vi "Dust_Type_Menu.vi"(8 "error in (no error)":errorcluster, 10 "Small?":bool, 11 "Enable":bool=TRUE) -> (0 "error out":errorcluster, 1 "Action Taken":T6(ring), 2 "Dust Properties":T3, 3 "Dust Info":T4 {"Batch" step=1; "Type" step=1; "Dust Source Builder:" items=["Keith Drake", "Nick Beaty", "Anthony Shu", "David James", "John Fontanese"]})   [LabVIEW 2013]
doc: "Displays a standard dialog box that prompts users to enter information, such as a user name and password.\n--------------------\n\nThis Express VI is configured as follows:\n\nMessage to Display to the User:Please Enter Experiment Settings Information For Database Storage.\nThe inputs are: \nNumber: Please Enter Group ID\nText Entry Box: Please Enter Tags:\nText Entry Box: Please Enter Experiment Description:"
uses:
  <vilib>/Utility/miscctls.llb/LVPointTypeDef.ctl
  <vilib>/addons/database/_DB Variant To Data/Database Variant To Data.xnode
  Controls/source_builders.ctl
  <userlib>/_OpenG.lib/array/array.llb/Remove Duplicates from 1D Array (String)__ogtk.vi
  <userlib>/_OpenG.lib/array/array.llb/Search 1D Array (String)__ogtk.vi
  <userlib>/_OpenG.lib/array/array.llb/Index 1D Array Elements (String)__ogtk.vi
  Controls/dust type.ctl
  Controls/dust_type_indicator.ctl
  Controls/Dust_list.ctl
panel:
  out "Query in Standard Format":string
  out "Maxes Array":T1(array[cluster])
  out "All Dust Types":T2[](array[typedef])
  in  "Transfer":bool caption="OK2"
  in  "Controls":T4 {"Batch" min=1 max=2 step=1; "Type" min=1 max=10 step=1; "Dust Source Builder:" items=["Keith Drake", "Nick Beaty", "Anthony Shu", "David James", "John Fontanese"]}
  in  "Create New":bool caption="OK2"
  in  "Cancel":bool
  in  "Update":bool caption="OK1"
  # "Please Enter Dust Information For Storage in the CCLDAS Database."
  # "Dust Information"
  # "Dust Information"
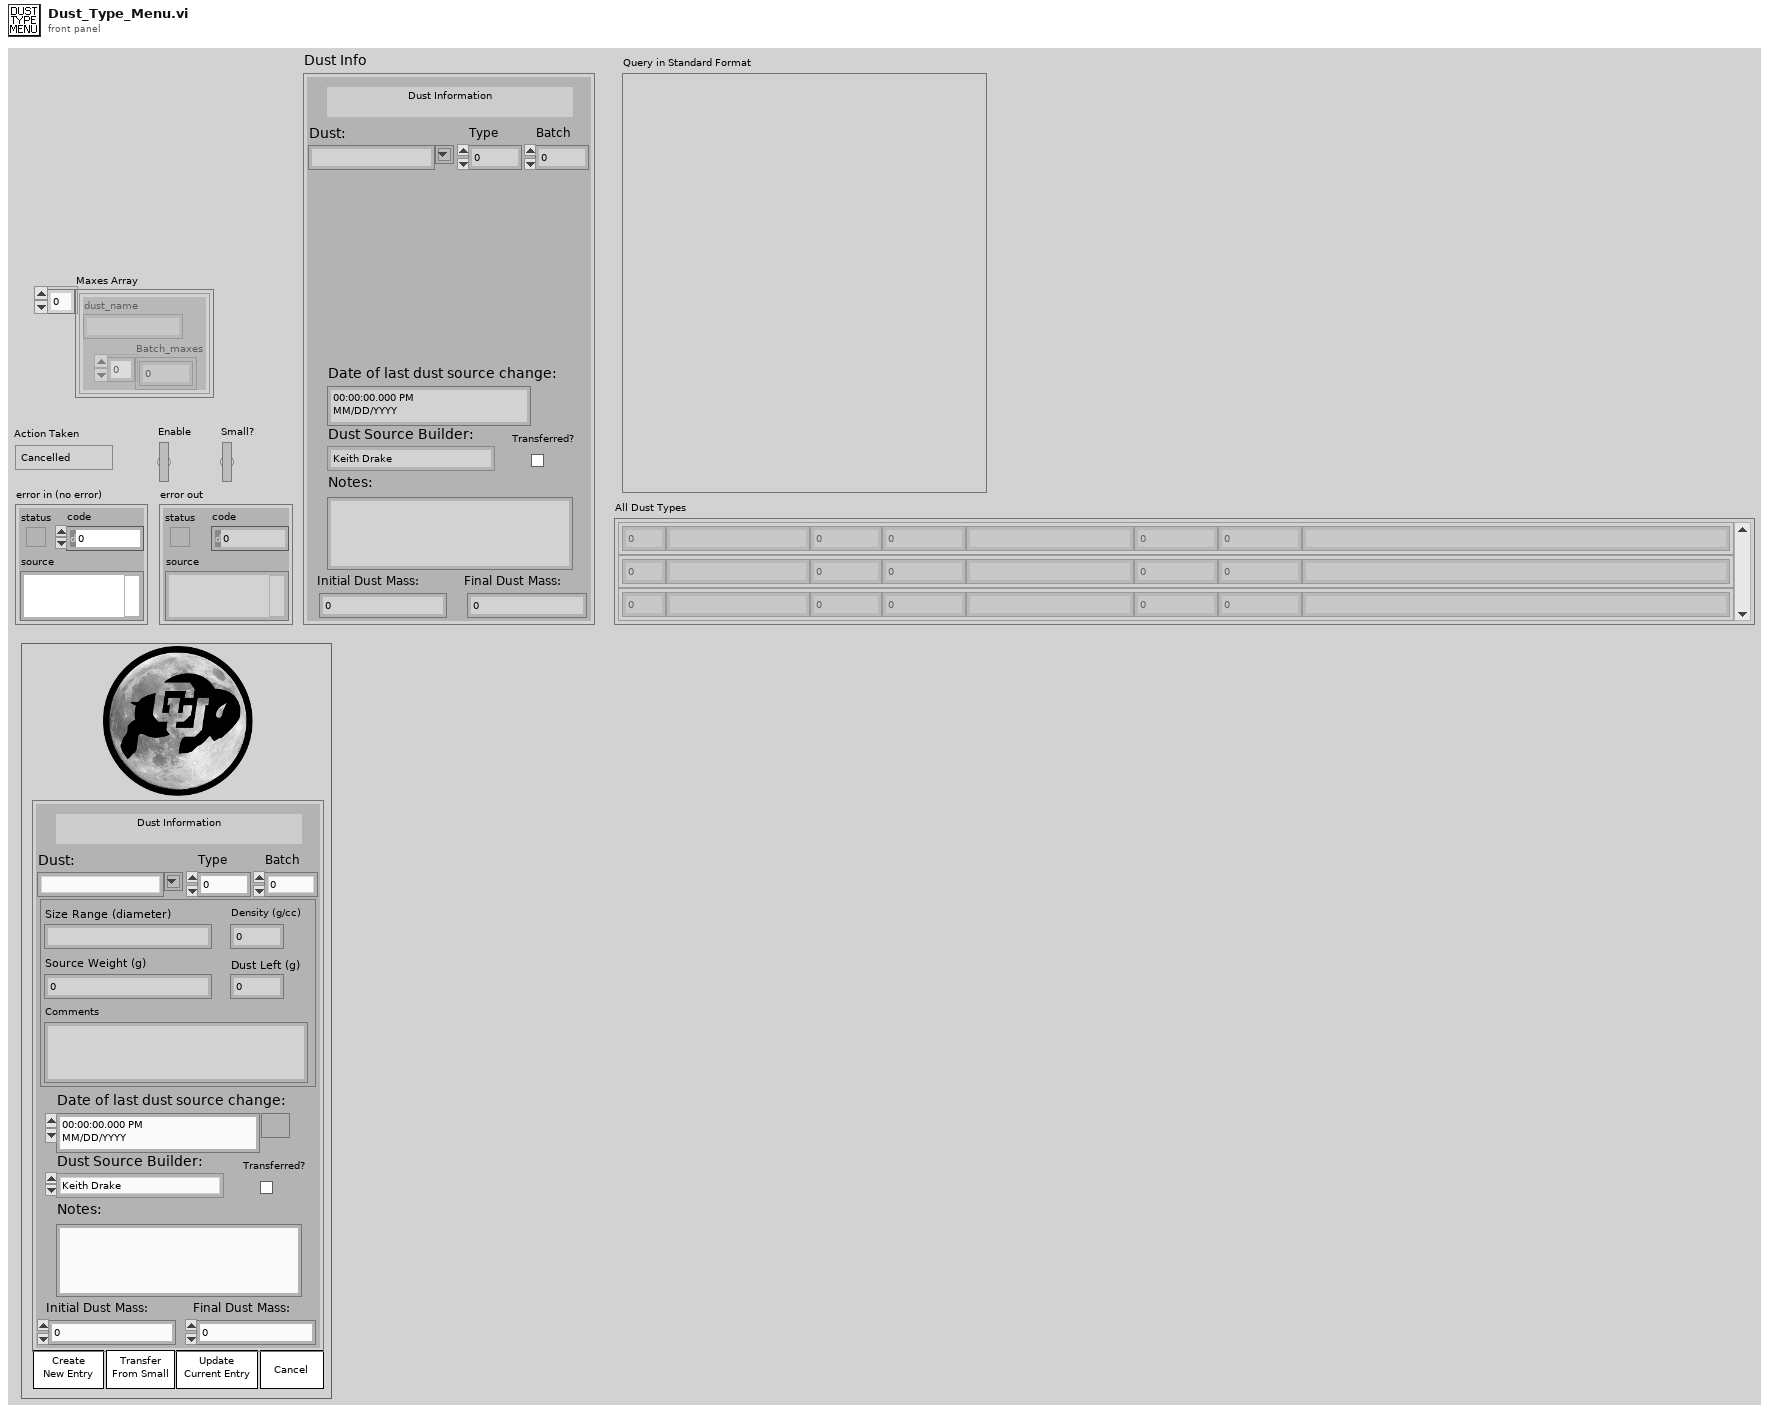
[diagram p1: front panel]
types:
  T1 = cluster{"dust_name":string, "Batch_maxes":i32[]}[]
  T2 = typedef "dust_list.ctl" = cluster{"id_dust_type":i32, "dust_name":string, "dust_density":dbl, "source_weight":dbl, "size":string, "bottle_weight":dbl, "dust_mass":dbl, "comments":string}
  T3 = typedef "dust_type_indicator.ctl" = cluster{"id_dust_type":i32, "Size Range (diameter)":string, "Density (g/cc)":dbl, "Source Weight (g)":dbl, "Dust Left (g)":dbl, "Comments":string}
  T4 = typedef "dust type.ctl" = cluster{"Dust info id":u16, "Integer Timestamp":i64, "Dust:":string, "Dust Source Builder:":T5, "Notes:":string, "Date of last dust source change:":timestamp, "Initial Dust Mass:":dbl, "Final Dust Mass:":dbl, "Type":u16, "Batch":u16, "dust type id":u16, "Transferred?":bool}
  T5 = typedef "source_builders.ctl" = u16
  T6 = enum16{"Cancelled", "New", "Updated", "Transferred"}
  T7 = enum8{"Enabled", "Disabled", "Disabled and Grayed Out"}
  T8 = typedef "LVPointTypeDef.ctl" = cluster{"Horizontal":i16, "Vertical":i16}
  T9 = enum16{"dust_name", "dust_density", "source_weight", "bottle_weight", "dust_weight"}
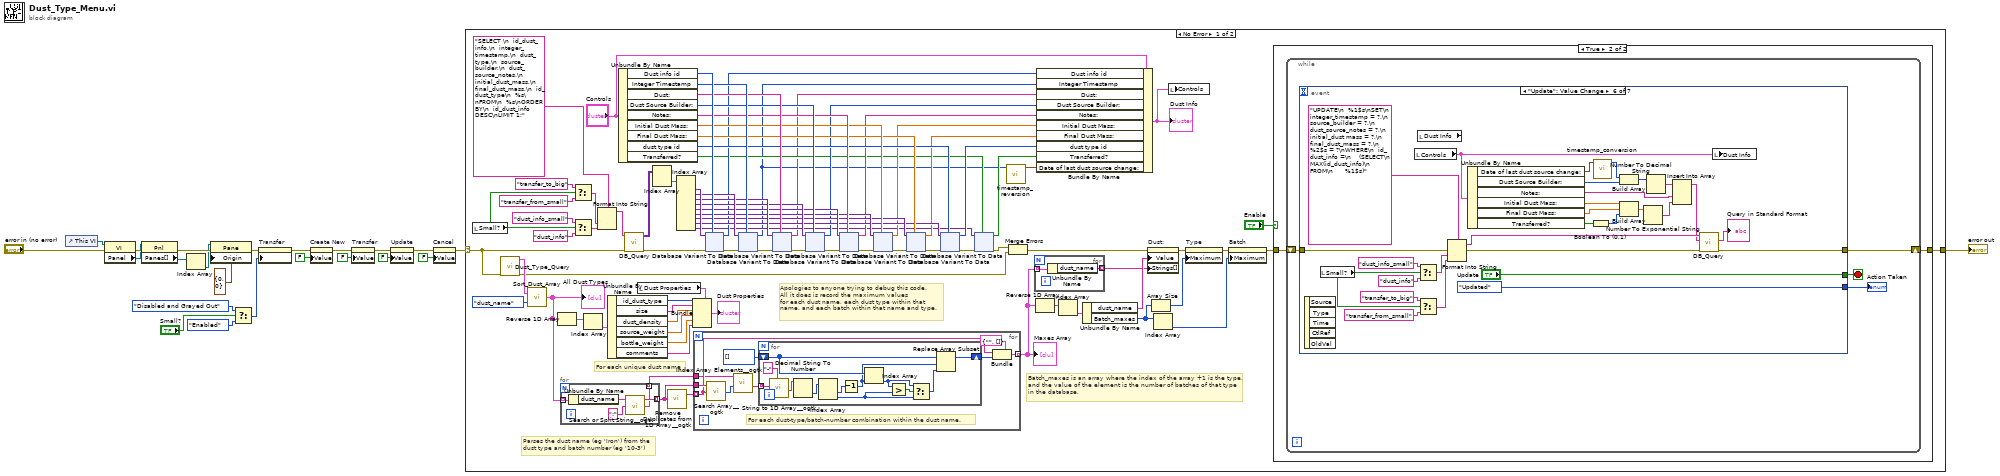
[diagram p0: block diagram]
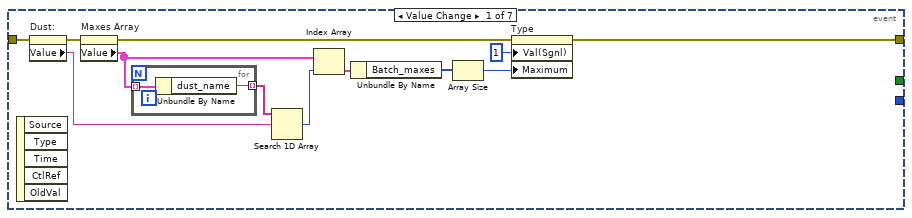
[diagram p3: hidden frame]
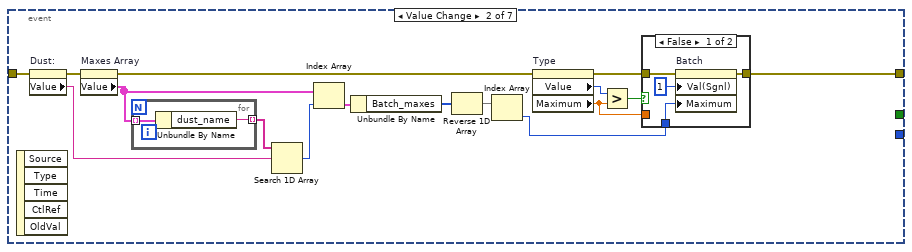
[diagram p4: hidden frame]
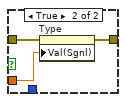
[diagram p5: hidden frame]
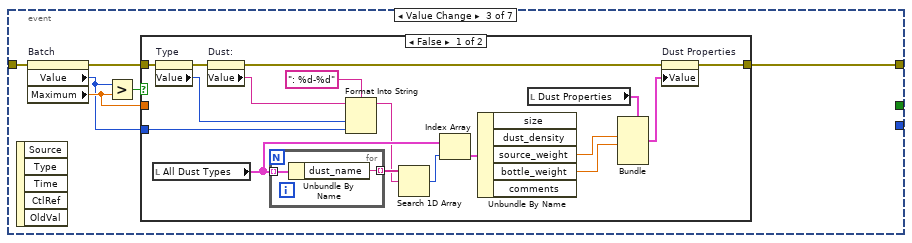
[diagram p6: hidden frame]
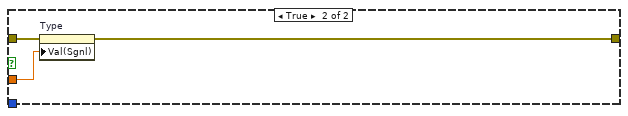
[diagram p7: hidden frame]
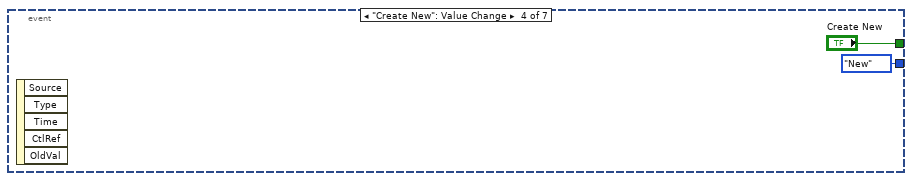
[diagram p8: hidden frame]
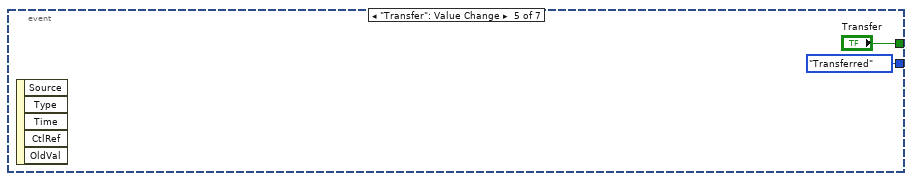
[diagram p9: hidden frame]
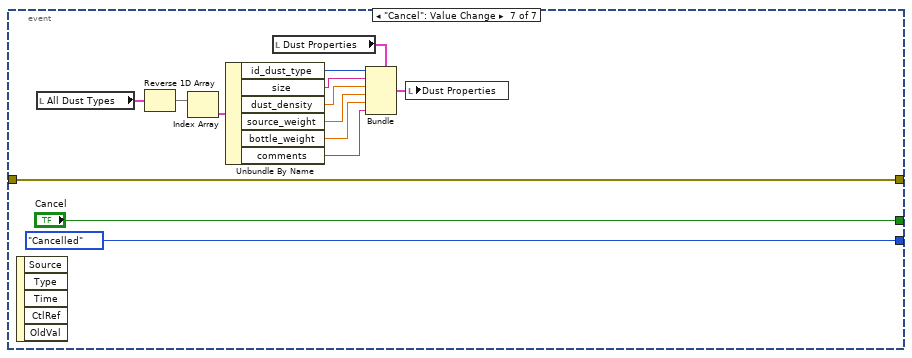
[diagram p10: hidden frame]
diagram:
  n1 = control-ref of="This VI"() -> (w22:refnum<vi>)
  n2 = property class="VI"(reference=w22, error in="error in (no error)") -> (error out=w21:errorcluster, "Panel"=w20:refnum<vi>)  [unwired: 1 out]
  n3 = property class="Pnl"(reference=w20, error in=w21) -> (error out=w19:errorcluster, "Panes[]"=w18:refnum<vi>[])  [unwired: 1 out]
  n4 = Index Array(array=w18) -> (element=w17:refnum<vi>)  [unwired: 1 in]
  n5 = property class="Pane"(reference=w17, error in=w19, "Origin"=T8 {"Horizontal"=0, "Vertical"=0}) -> (error out=w10:errorcluster)  [unwired: 1 out]
  n6 = Select(t=T7."Disabled and Grayed Out" ("Disabled"), s="Small?", f=T7."Enabled" ("Disabled")) -> (s? t:f=w13:T7)
  n7 = property on="Transfer" class="Bool (strict)"(error in=w10, "DisabledEnum"=w13) -> (error out=w5:errorcluster)  [unwired: 1 in, 1 out]
  n8 = property on="Create New" class="Bool (strict)"(error in=w5, "Value"=FALSE ("Create New")) -> (error out=w7:errorcluster)  [unwired: 1 in, 1 out]
  n9 = property on="Transfer" class="Bool (strict)"(error in=w7, "Value"=FALSE ("Transfer")) -> (error out=w9:errorcluster)  [unwired: 1 in, 1 out]
  n10 = property on="Update" class="Bool (strict)"(error in=w9, "Value"=FALSE ("Update")) -> (error out=w8:errorcluster)  [unwired: 1 in, 1 out]
  n11 = property on="Cancel" class="Bool (strict)"(error in=w8, "Value"=FALSE ("Cancel")) -> (error out=w6:errorcluster)  [unwired: 1 in, 1 out]
  n12 = case shown="No Error" w6 {
    selector: w6 -> [w58 w544]
    tunnel: [w35 w544] -> w23
    frame No Error {
      # "Batch_maxes is an array where the index of the array +1 is the type,\nand the value of the element is the number of batches of that type\nin the database."
      # "For each unique dust name"
      # "Parses the dust name (eg 'Iron') from the\ndust type and batch number (eg '10-3')"
      # "Apologies to anyone trying to debug this code.\nAll it does is record the maximum values\nfor each dust name, each dust type within that\nname, and each batch within that name and type."
      n13 = local read "Small?"() -> (w98:bool)
      n14 = call "Dust_Type_Query.vi"("error in (no error)"=w58) -> ("error out"=w52:errorcluster, "Dust Type Array"=w57:T2[])  [unwired: 9 in]
      n15 = call "Sort_Dust_Array.vi"("Order by..."=T9."dust_name", "Array In"=w57) -> ("Array out"=w53:T2[])
      "All Dust Types" <- w53
      n16 = Reverse 1D Array(array=w53) -> (reversed array=w47:T2[])
      n17 = for {
        tunnel: w53 -> [w255] mode=indexing
        tunnel: [w253] -> w49 mode=indexing
        tunnel: [w251] -> w50 mode=indexing
        n18 = Unbundle By Name(w255) -> ("dust_name"=w252:string)
        n19 = call <userlib>:"Search or Split String__ogtk.vi"("search string/char (-)"=":", "string"=w252) -> ("substring after match"=w251:string, "substring before match"=w253:string)  [unwired: 1 in, 1 out]
      }
      n20 = Select(t="transfer_to_big", s=w98, f="transfer_from_small") -> (s? t:f=w99:string)
      n21 = Select(t="dust_info_small", s=w98, f="dust_info") -> (s? t:f=w103:string)
      n22 = Index Array(array=w47) -> (element=w56:T2)  [unwired: 1 in]
      n23 = Format Into String(format string="SELECT \n  id_dust_info,\n  integer_timestamp,\n  dust_type,\n  source_builder,\n  dust_source_notes,\n  initial_dust_mass,\n  final_dust_mass,\n  id_dust_type\n  %s\nFROM\n  %s\nORDER BY\n  id_dust_info DESC\nLIMIT 1;" ("SQL query"), w99, w103) -> (resulting string=w102:string)  [unwired: 2 in, 1 out]
      n24 = Unbundle By Name(w56) -> ("id_dust_type"=w24:i32, "size"=w25:string, "dust_density"=w26:dbl, "source_weight"=w27:dbl, "bottle_weight"=w28:dbl, "comments"=w29:string)
      n25 = Unbundle By Name("Controls") -> ("Dust info id"=w93:u16, "Integer Timestamp"=w90:i64, "Dust:"=w87:string, "Dust Source Builder:"=w85:T5, "Notes:"=w82:string, "Initial Dust Mass:"=w79:dbl, "Final Dust Mass:"=w75:dbl, "dust type id"=w72:u16, "Transferred?"=w63:bool)
      n26 = call "DB_Query.vi"("error in (no error)"=w58, "Parameterized Query"=w102) -> ("error out"=w97:errorcluster, "Results"=w96:variant[][])  [unwired: 7 in, 1 out]
      n27 = local read "Dust Properties"() -> (w55:T3)
      n28 = Index Array(array=w96) -> (element=w95:variant[])  [unwired: 2 in]
      n29 = call-poly <userlib>:"Remove Duplicates from 1D Array__ogtk.vi"("Input Array"=w49) -> ("Output Array"=w51:string[])  [unwired: 1 out]
      n30 = Index Array(array=w95) -> (element #1=w94:variant, element #2=w91:variant, element #3=w88:variant, element #4=w84:variant, element #5=w81:variant, element #6=w78:variant, element #7=w76:variant, element #8=w73:variant, element #9=w61:variant)  [unwired: 9 in]
      n31 = Bundle(cluster=w55, "id_dust_type"=w24, "Size Range (diameter)"=w25, "Density (g/cc)"=w26, "Source Weight (g)"=w27, "Dust Left (g)"=w28, "Comments"=w29) -> (→"Dust Properties":T3)
      n32 = for {
        tunnel: w51 -> [w236] mode=indexing
        tunnel: w50 -> [w234]
        tunnel: w49 -> [w238]
        tunnel: [w230] -> w39 mode=indexing
        # "For each dust-type/batch-number combination within the dust name."
        n33 = call-poly <userlib>:"Search Array__ogtk.vi"("Array"=w238, "Element Data"=w236) -> ("Indices of Elements"=w235:i32[])  [unwired: 7 in]
        n34 = call-poly <userlib>:"Index Array Elements__ogtk.vi"("indices"=w235, "array"=w234) -> ("elements"=w233:string[])  [unwired: 9 in]
        n35 = for {
          tunnel: w233 -> [w247] mode=indexing
          shift-right: [w245] -> w231
          shift-left: i32[] [] ("array") -> [w244]
          n36 = call <userlib>:"String to 1D Array__ogtk.vi"("delimiter (Tab)"="-", "string"=w247) -> ("Array of Strings"=w249:string[])  [unwired: 9 in]
          n37 = Decimal String To Number(string=w249) -> (number=w248:i32[])  [unwired: 2 in, 1 out]
          n38 = Index Array(array=w248) -> (element #1=w246:i32, element #2=w240:i32)  [unwired: 2 in]
          n39 = Decrement(x=w246) -> (x-1=w243:i32)
          n40 = Index Array(array=w244, index=w243) -> (element=w241:i32)
          n41 = Greater?(x=w241, y=w240) -> (0:w242:bool)
          n42 = Select(t=w241, s=w242, f=w240) -> (s? t:f=w239:i32)
          n43 = Replace Array Subset(array=w244, new element=w239, index=w243) -> (w245:i32[])
        }
        n44 = Bundle(cluster=cluster{"dust_name":string, "Batch_maxes":i32[]} {"dust_name"="", "Batch_maxes"=[]}, "dust_name"=w236, "Batch_maxes"=w231) -> (w230:cluster{"dust_name":string, "Batch_maxes":i32[]})
      }
      "Maxes Array" <- w39
      n45 = xnode "Database Variant To Data"("database variant"=w94, "error in (no error)"=w97, "type"=w93) -> ("data"=w70:u16, "error out"=w92:errorcluster)
      n46 = xnode "Database Variant To Data"("database variant"=w91, "error in (no error)"=w92, "type"=w90) -> ("data"=w30:i64, "error out"=w89:errorcluster)
      n47 = xnode "Database Variant To Data"("database variant"=w88, "error in (no error)"=w89, "type"=w87) -> ("data"=w32:string, "error out"=w86:errorcluster)
      n48 = xnode "Database Variant To Data"("database variant"=w84, "error in (no error)"=w86, "type"=w85) -> ("data"=w69:T5, "error out"=w83:errorcluster)
      n49 = xnode "Database Variant To Data"("database variant"=w81, "error in (no error)"=w83, "type"=w82) -> ("data"=w68:string, "error out"=w80:errorcluster)
      n50 = xnode "Database Variant To Data"("database variant"=w78, "error in (no error)"=w80, "type"=w79) -> ("data"=w67:dbl, "error out"=w77:errorcluster)
      n51 = xnode "Database Variant To Data"("database variant"=w76, "error in (no error)"=w77, "type"=w75) -> ("data"=w66:dbl, "error out"=w74:errorcluster)
      n52 = xnode "Database Variant To Data"("database variant"=w73, "error in (no error)"=w74, "type"=w72) -> ("data"=w65:u16, "error out"=w64:errorcluster)
      n53 = xnode "Database Variant To Data"("database variant"=w61, "error in (no error)"=w64, "type"=w63) -> ("data"=w62:bool, "error out"=w60:errorcluster)
      n54 = call "timestamp_reversion.vi"("Integer Timestamp"=w30) -> ("time stamp"=w31:timestamp)  [unwired: 8 in, 1 out]
      n55 = Merge Errors(w60, w52) -> (w41:errorcluster)
      n56 = for {
        tunnel: w39 -> [w229] mode=indexing
        tunnel: [w228] -> w38 mode=indexing
        n57 = Unbundle By Name(w229) -> ("dust_name"=w228:string)
      }
      n58 = Reverse 1D Array(array=w39) -> (reversed array=w37:T1)
      n59 = Bundle By Name(cluster="Controls", "Dust info id"=w70, "Integer Timestamp"=w30, "Dust:"=w32, "Dust Source Builder:"=w69, "Notes:"=w68, "Initial Dust Mass:"=w67, "Final Dust Mass:"=w66, "dust type id"=w65, "Transferred?"=w62, "Date of last dust source change:"=w31) -> (w34:T4)
      "Dust Info" <- w34
      n60 = Index Array(array=w37) -> (element=w48:cluster{"dust_name":string, "Batch_maxes":i32[]})  [unwired: 1 in]
      n61 = Unbundle By Name(w48) -> ("dust_name"=w42:string, "Batch_maxes"=w46:i32[])
      n62 = property on="Dust:" class="CmbBox"(error in=w41, "Value"=w42, "Strings[]"=w38) -> (error out=w40:errorcluster)  [unwired: 1 in, 1 out]
      n63 = Array Size(array=w46) -> (size(s)=w45:i32)
      n64 = Index Array(array=w46) -> (element=w44:i32)  [unwired: 1 in]
      n65 = local write "Controls"(w34) -> ()
      n66 = property on="Type" class="DigNum (strict)"(error in=w40, "Maximum"=w45) -> (error out=w43:errorcluster)  [unwired: 1 in, 1 out]
      n67 = property on="Batch" class="DigNum (strict)"(error in=w43, "Maximum"=w44) -> (error out=w36:errorcluster)  [unwired: 1 in, 1 out]
      n68 = case shown="True" "Enable" {
        tunnel: w36 -> [w107 w109]
        tunnel: [w107 w108] -> w35
        frame False {
        }
        frame True {
          n69 = while {
            shift-right: [w112] -> w108
            shift-left: w109 -> [w113]
            stop <- w111 stop-if-true
            n70 = event shown="[5] \"Update\": Value Change" {
              selector: _ -> [_ _ _ _ _ _ _]
              dyn-events: _ -> [_ _ _ _ _ _ _]
              timeout: _ -> [_ _ _ _ _ _ _]
              tunnel: w113 -> [w125 w137 w155 _ _ w203 w226]
              tunnel: [w114 w131 w154 _ _ w187 w226] -> w112
              tunnel: [_ _ _ "Create New" "Transfer" "Update" "Cancel"] -> w111
              tunnel: [_ _ _ T6."New" ("Action Taken") T6."Transferred" ("Action Taken") T6."Updated" ("Action Taken") T6."Cancelled" ("Action Taken")] -> w110
              event Value Change {
                n71 = event-data() -> ()  [unwired: 1 in, 5 out]
                n72 = property on="Dust:" class="CmbBox"(error in=w125) -> (error out=w124:errorcluster, "Value"=w115:string)  [unwired: 1 in, 1 out]
                n73 = property on="Maxes Array" class="Arr (strict)"(error in=w124) -> (error out=w123:errorcluster, "Value"=w120:T1)  [unwired: 1 in, 1 out]
                n74 = for {
                  tunnel: w120 -> [w127] mode=indexing
                  tunnel: [w126] -> w122 mode=indexing
                  n75 = Unbundle By Name(w127) -> ("dust_name"=w126:string)
                }
                n76 = Search 1D Array(1D array=w122, element=w115) -> (index of element=w116:i32)  [unwired: 1 in]
                n77 = Index Array(array=w120, index=w116) -> (element=w119:cluster{"dust_name":string, "Batch_maxes":i32[]})
                n78 = Unbundle By Name(w119) -> ("Batch_maxes"=w118:i32[])
                n79 = Array Size(array=w118) -> (size(s)=w117:i32)
                n80 = property on="Type" class="DigNum (strict)"(error in=w123, "Val(Sgnl)"=u16 1 ("Value"), "Maximum"=w117) -> (error out=w114:errorcluster)  [unwired: 1 in, 1 out]
              }
              event Value Change {
                n81 = event-data() -> ()  [unwired: 1 in, 5 out]
                n82 = property on="Dust:" class="CmbBox"(error in=w137) -> (error out=w143:errorcluster, "Value"=w141:string)  [unwired: 1 in, 1 out]
                n83 = property on="Maxes Array" class="Arr (strict)"(error in=w143) -> (error out=w128:errorcluster, "Value"=w139:T1)  [unwired: 1 in, 1 out]
                n84 = for {
                  tunnel: w139 -> [w152] mode=indexing
                  tunnel: [w151] -> w142 mode=indexing
                  n85 = Unbundle By Name(w152) -> ("dust_name"=w151:string)
                }
                n86 = Search 1D Array(1D array=w142, element=w141) -> (index of element=w140:i32)  [unwired: 1 in]
                n87 = Index Array(array=w139, index=w140) -> (element=w138:cluster{"dust_name":string, "Batch_maxes":i32[]})
                n88 = Unbundle By Name(w138) -> ("Batch_maxes"=w136:i32[])
                n89 = Reverse 1D Array(array=w136) -> (reversed array=w135:i32[])
                n90 = Index Array(array=w135) -> (element=w129:i32)  [unwired: 1 in]
                n91 = property on="Type" class="DigNum (strict)"(error in=w128) -> (error out=w133:errorcluster, "Value"=w134:u16, "Maximum"=w132:dbl)  [unwired: 1 in, 1 out]
                n92 = Greater?(x=w134, y=w132) -> (0:w130:bool)
                n93 = case shown="False" w130 {
                  tunnel: w133 -> [w146 w150]
                  tunnel: w132 -> [_ w149]
                  tunnel: [w145 w148] -> w131
                  tunnel: w129 -> [w144 _]
                  frame False {
                    n94 = property on="Batch" class="DigNum (strict)"(error in=w146, "Val(Sgnl)"=u16 1 ("Value (Signaling)"), "Maximum"=w144) -> (error out=w145:errorcluster)  [unwired: 1 in, 1 out]
                  }
                  frame True {
                    n95 = property on="Type" class="DigNum (strict)"(error in=w150, "Val(Sgnl)"=w149) -> (error out=w148:errorcluster)  [unwired: 1 in, 1 out]
                  }
                }
              }
              event Value Change {
                n96 = event-data() -> ()  [unwired: 1 in, 5 out]
                n97 = property on="Batch" class="DigNum (strict)"(error in=w155) -> (error out=w158:errorcluster, "Value"=w153:u16, "Maximum"=w157:dbl)  [unwired: 1 in, 1 out]
                n98 = Greater?(x=w153, y=w157) -> (0:w156:bool)
                n99 = case shown="False" w156 {
                  tunnel: w158 -> [w164 w180]
                  tunnel: w157 -> [_ w179]
                  tunnel: [w159 w178] -> w154
                  tunnel: w153 -> [w163 _]
                  frame False {
                    n100 = local read "All Dust Types"() -> (w170:T2[])
                    n101 = property on="Type" class="DigNum (strict)"(error in=w164) -> (error out=w165:errorcluster, "Value"=w161:u16)  [unwired: 1 in, 1 out]
                    n102 = property on="Dust:" class="CmbBox"(error in=w165) -> (error out=w160:errorcluster, "Value"=w162:string)  [unwired: 1 in, 1 out]
                    n103 = for {
                      tunnel: w170 -> [w177] mode=indexing
                      tunnel: [w176] -> w169 mode=indexing
                      n104 = Unbundle By Name(w177) -> ("dust_name"=w176:string)
                    }
                    n105 = Format Into String(format string=": %d-%d", initial string=w162, w161, w163) -> (resulting string=w166:string)  [unwired: 1 in, 1 out]
                    n106 = Search 1D Array(1D array=w169, element=w166) -> (index of element=w168:i32)  [unwired: 1 in]
                    n107 = Index Array(array=w170, index=w168) -> (element=w172:T2)
                    n108 = Unbundle By Name(w172) -> ("source_weight"=w174:dbl, "bottle_weight"=w175:dbl)  [unwired: 3 out]
                    n109 = local read "Dust Properties"() -> (w173:T3)
                    n110 = Bundle(cluster=w173, "Density (g/cc)"=w174, "Source Weight (g)"=w175) -> (w171:T3)  [unwired: 4 in]
                    n111 = property on="Dust Properties" class="Clust (strict)"(error in=w160, "Value"=w171) -> (error out=w159:errorcluster)  [unwired: 1 in, 1 out]
                  }
                  frame True {
                    n112 = property on="Type" class="DigNum (strict)"(error in=w180, "Val(Sgnl)"=w179) -> (error out=w178:errorcluster)  [unwired: 1 in, 1 out]
                  }
                }
              }
              event "Create New": Value Change {
                n113 = event-data() -> ()  [unwired: 1 in, 5 out]
              }
              event "Transfer": Value Change {
                n114 = event-data() -> ()  [unwired: 1 in, 5 out]
              }
              event "Update": Value Change {
                n115 = event-data() -> ()  [unwired: 1 in, 5 out]
                n116 = local read "Small?"() -> (w209:bool)
                n117 = local read "Controls"() -> (w185:T4)
                n118 = local read "Dust Info"() -> ()  [unwired: 1 out]
                n119 = Select(t="dust_info_small", s=w209, f="dust_info") -> (s? t:f=w205:string)
                n120 = Select(t="transfer_to_big", s=w209, f="transfer_from_small") -> (s? t:f=w204:string)
                n121 = Format Into String(format string="UPDATE\n  %1$s\nSET\n  integer_timestamp = ?,\n  source_builder = ?,\n  dust_source_notes = ?,\n  initial_dust mass = ?,\n  final_dust_mass = ?,\n  %2$s = ?\nWHERE\n  id_dust_info =\n    (SELECT\n      MAX(id_dust_info)\n    FROM\n      %1$s)", error in=w203, w205, w204) -> (resulting string=w211:string, error out=w202:errorcluster)  [unwired: 1 in]
                n122 = Unbundle By Name(w185) -> ("Date of last dust source change:"=w201:timestamp, "Dust Source Builder:"=w198:T5, "Notes:"=w191:string, "Initial Dust Mass:"=w196:dbl, "Final Dust Mass:"=w195:dbl, "Transferred?"=w200:bool)
                n123 = Boolean To (0,1)(Boolean=w200) -> (0, 1=w194:i16)
                n124 = call "timestamp_conversion.vi"("Time Stamp"=w201) -> ("Integer Time"=w199:i64)  [unwired: 8 in, 1 out]
                n125 = Build Array(w199, w198) -> (w197:i64[])
                n126 = Build Array(w196, w195, w194) -> (w193:dbl[])
                n127 = Number To Exponential String(number=w193) -> (E-format string=w190:string[])  [unwired: 3 in]
                n128 = Number To Decimal String(number=w197) -> (decimal integer string=w192:string[])  [unwired: 1 in]
                n129 = Insert Into Array(array=w192, new element #1=w191, new element #2=w190) -> (w189:string[])  [unwired: 1 in]
                n130 = call "DB_Query.vi"("error in (no error)"=w202, "Parameters"=w189, "Parameterized Query"=w211) -> ("error out"=w187:errorcluster, "Query in Standard Format"=→"Query in Standard Format":string)  [unwired: 6 in, 1 out]
                n131 = local write "Dust Info"(w185) -> ()
              }
              event "Cancel": Value Change {
                n132 = event-data() -> ()  [unwired: 1 in, 5 out]
                n133 = local read "All Dust Types"() -> (w223:T2[])
                n134 = Reverse 1D Array(array=w223) -> (reversed array=w225:T2[])
                n135 = Index Array(array=w225) -> (element=w224:T2)  [unwired: 1 in]
                n136 = Unbundle By Name(w224) -> ("id_dust_type"=w214:i32, "size"=w215:string, "dust_density"=w216:dbl, "source_weight"=w217:dbl, "bottle_weight"=w218:dbl, "comments"=w219:string)
                n137 = local read "Dust Properties"() -> (w222:T3)
                n138 = Bundle(cluster=w222, "id_dust_type"=w214, "Size Range (diameter)"=w215, "Density (g/cc)"=w216, "Source Weight (g)"=w217, "Dust Left (g)"=w218, "Comments"=w219) -> (w221:T3)
                n139 = local write "Dust Properties"(w221) -> ()
              }
            }
            "Action Taken" <- w110
          }
        }
      }
    }
    frame Error {
    }
  }
  "error out" <- w23
